vi "SimpleConnectAndSubscribe.vi"() -> ()   [LabVIEW 2016, in "AWS_IoT.lvlib"]
doc: "A basic client example that connects to a server, subscribes to a variety of topics and receives responses for the topics. \n\n© 2015 - daq.io, LLC - Peter Adelhardt"
uses:
  AWS_IoT.lvlib
  MQTT/Controls/QoS.ctl
  MQTT/Controls/MessageType.ctl
  MQTT/Controls/Connection_Return_Codes.ctl
  Controls/certs.ctl
  MQTT/Controls/ConnectMeta.ctl
  MQTT/Controls/Retain_Flag.ctl
  MQTT/Controls/DUP_Flag.ctl
  MQTT/Controls/Connect_Flags.ctl
panel:
  in  "cert path":T1={"client cert file"=path "", "CA file"=path "", "client key file"=path ""}
  out "Connection Status":T2=enum."Connection refused: not authorized"
  out "Messages":T4(array[cluster])
  in  "Stop Reading":bool
  in  "MQTT Broker":cluster{"address (IP)":string, "port":u16}={"address (IP)"="a28e3t2sj3ekjh.iot.us-west-2.amazonaws.com", "port"=8883}
  in  "Subscription Info Array":cluster{"Topic":string, "QoS":T5}[](array[cluster])=[{"Topic"="testtopic/LVMQTT", "QoS"=enum."At most once"}]
  out "Granted QoS Levels":T5[](array[typedef])
  in  "Client ID":string="LVSubscribeClient"
  out "error out":errorcluster
  in  "error in (no error)":errorcluster
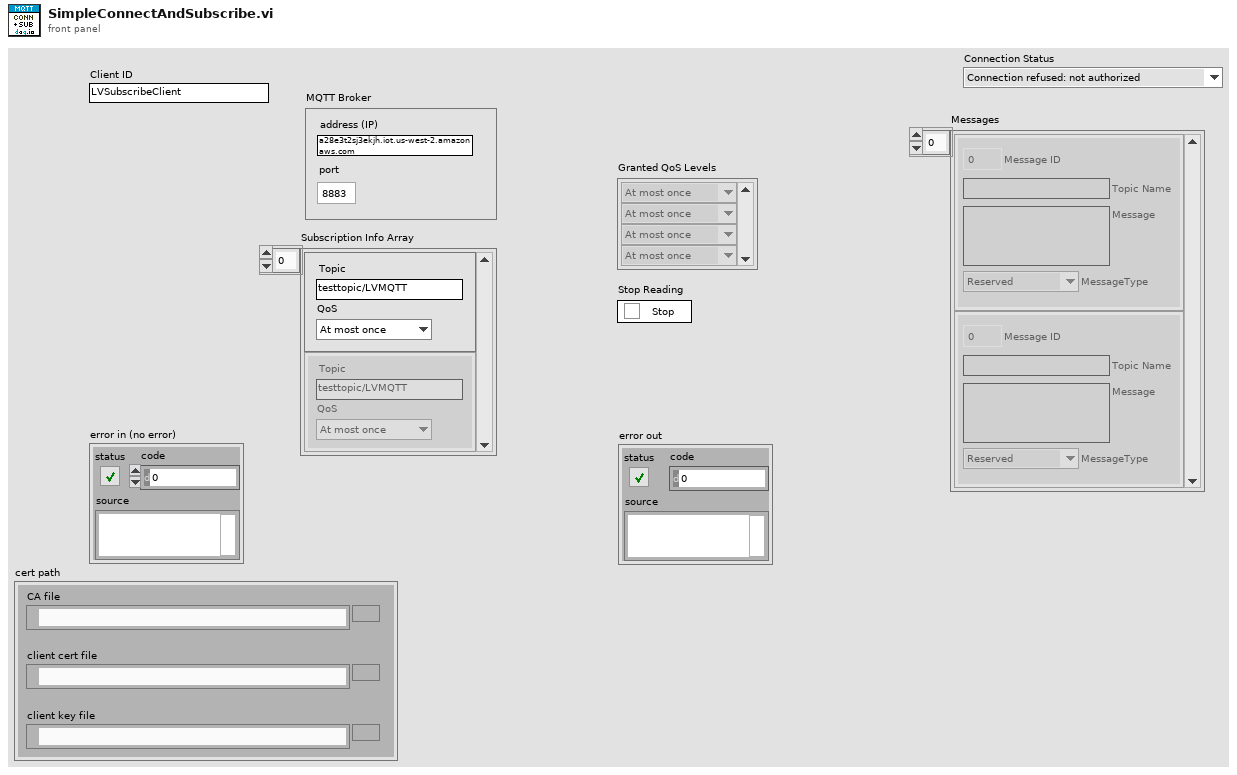
[diagram p1: front panel]
types:
  T1 = typedef "AWS_IoT.lvlib/certs.ctl" = cluster{"client cert file":path, "CA file":path, "client key file":path}
  T2 = typedef "AWS_IoT.lvlib/Connection_Return_Codes.ctl" = enum16{"Connection accepted", "Connection refused: unacceptable protocol version", "Connection refused: identifier rejected", "Connection refused: Server unavailable", "Connection refused: bad user name or password", "Connection refused: not authorized"}
  T3 = typedef "AWS_IoT.lvlib/MessageType.ctl" = enum32{"Reserved", "CONNECT", "CONNACK", "PUBLISH", "PUBACK", "PUBREC", "PUBREL", "PUBCOMP", "SUBSCRIBE", "SUBACK", "UNSUBSCRIBE", "UNSUBACK", "PINGREQ", "PINGRESP", "DISCONNECT", "Reserved2"}
  T4 = cluster{"Message ID":u16, "Topic Name":string, "Message ":string, "MessageType":T3}[]
  T5 = typedef "AWS_IoT.lvlib/QoS.ctl" = enum8{"At most once", "At least once", "Exactly once", "Reserved"}
  T6 = cluster{"Message ID":u16, "Topic Name":string, "Message":string, "MessageType":T3}
  T7 = typedef "AWS_IoT.lvlib/Connect_Flags.ctl" = cluster{"user name":bool, "password":bool, "will retain":bool, "will flag":bool, "clean session":bool, "reserved":bool, "will QoS":T5}
  T8 = typedef "AWS_IoT.lvlib/ConnectMeta.ctl" = cluster{"Retain":T9, "DUP":T10, "Keep Alive (sec)":u16, "QoS":T5}
  T9 = typedef "AWS_IoT.lvlib/Retain_Flag.ctl" = bool
  T10 = typedef "AWS_IoT.lvlib/DUP_Flag.ctl" = bool
  T11 = typedef "AWS_IoT.lvlib/SSL_Connection.ctl" = cluster{"connection ID":refnum<k5>, "TLS":cluster{"CXT ptr":i32, "SSL ptr":i32, "Socket ptr":i32}, "NIssleay library path":path, "server url":string}
  T12 = cluster{"Message ID":u16, "Topic Name":string, "Message":string, "MessageType":T3}[]
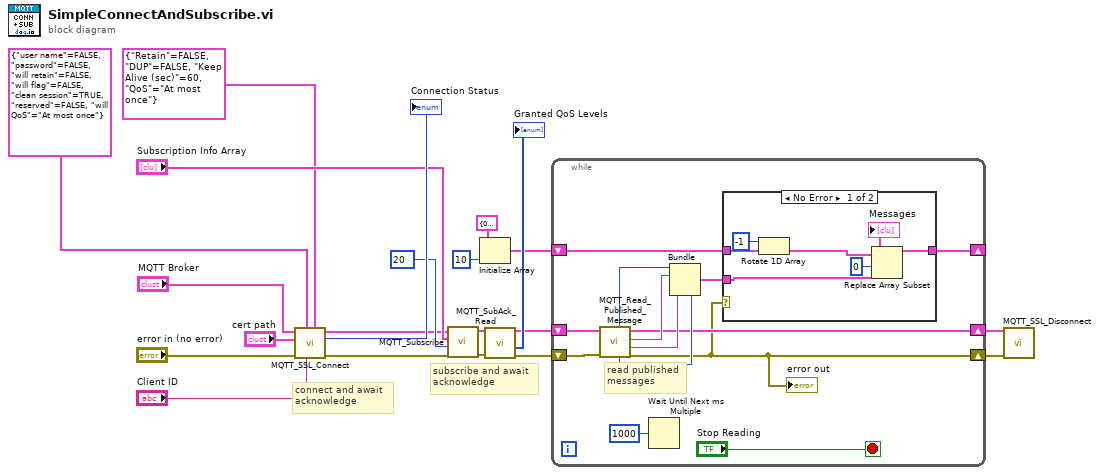
[diagram p0: block diagram]
diagram:
  # "connect and await\nacknowledge"
  # "subscribe and await\nacknowledge"
  n1 = call "MQTT_SSL_Connect.vi"("Connect Meta"=T8 {"Retain"=FALSE, "DUP"=FALSE, "Keep Alive (sec)"=60, "QoS"=enum."At most once"}, "Client ID"="Client ID", "Connect Flags"=T7 {"user name"=FALSE, "password"=FALSE, "will retain"=FALSE, "will flag"=FALSE, "clean session"=TRUE, "reserved"=FALSE, "will QoS"=enum."At most once"}, "error in (no error)"="error in (no error)", "cert path"="cert path", "MQTT Broker"="MQTT Broker") -> ("error out"=w10:errorcluster, "Connection Status"=→"Connection Status":T2, "SSL_Connection"=w9:T11)  [unwired: 3 in]
  n2 = call "MQTT_Subscribe.vi"("error in (no error)"=w10, "Message ID"=u16 20, "Subscription Info Array"="Subscription Info Array", "SSL_Connection"=w9) -> ("error out"=w13:errorcluster, "SSL_Connection"=w8:T11)  [unwired: 6 in]
  n3 = Initialize Array(T6 {"Message ID"=0, "Topic Name"="", "Message"="", "MessageType"=enum."Reserved"}, 10 ("dimension size")) -> (w1:T12)
  n4 = call "MQTT_SubAck_Read.vi"("error in (no error)"=w13, "SSL_Connection"=w8) -> ("error out"=w18:errorcluster, "Granted QoS Levels"=→"Granted QoS Levels":T5[], "SSL_Connection 2"=w17:T11)  [unwired: 7 in]
  n5 = while {
    shift-right: [w31] -> _
    shift-left: w1 -> [w33]
    shift-right: [w22] -> w16
    shift-left: w18 -> [w29]
    shift-right: [w24] -> w7
    shift-left: w17 -> [w30]
    stop <- "Stop Reading" stop-if-true
    # "read published\nmessages"
    n6 = call "MQTT_Read_Published_Message.vi"("error in (no error)"=w29, "SSL_Connection"=w30) -> ("error out"=w22:errorcluster, "Message"=w28:string, "Topic Name"=w27:string, "SSL_Connection"=w24:T11, "MessageType"=w25:T3, "Message ID"=w26:u16)  [unwired: 4 in]
    "error out" <- w22
    n7 = Wait Until Next ms Multiple(millisecond multiple=u32 1000) -> ()  [unwired: 1 out]
    n8 = Bundle("Message ID"=w26, "Topic Name"=w27, "Message"=w28, "MessageType"=w25) -> (w32:T6)  [unwired: 1 in]
    n9 = case shown="No Error" w22 {
      tunnel: w33 -> [w40 w41]
      tunnel: w32 -> [w38 _]
      tunnel: [w39 w41] -> w31
      frame No Error {
        n10 = Rotate 1D Array(1:w40, 2:-1 ("n")) -> (0:w36:T12)
        n11 = Replace Array Subset(array=w36, new element=w38, index=0) -> (w39:T12)
        "Messages" <- w39
      }
      frame Error {
      }
    }
  }
  n12 = call "MQTT_SSL_Disconnect.vi"("error in (no error)"=w16, "SSL_Connection"=w7) -> ()  [unwired: 9 in, 1 out]
